vi "Excel Step Content test.vi"() -> ()   [LabVIEW 2019]
uses:
  Ctrl/ProjectStepSelect.ctl
  Global/Process Global.vi
panel:
  out "error out":errorcluster
  out "receive string":string
  out "concatenated string":string
  out "step content":string[](array[string])
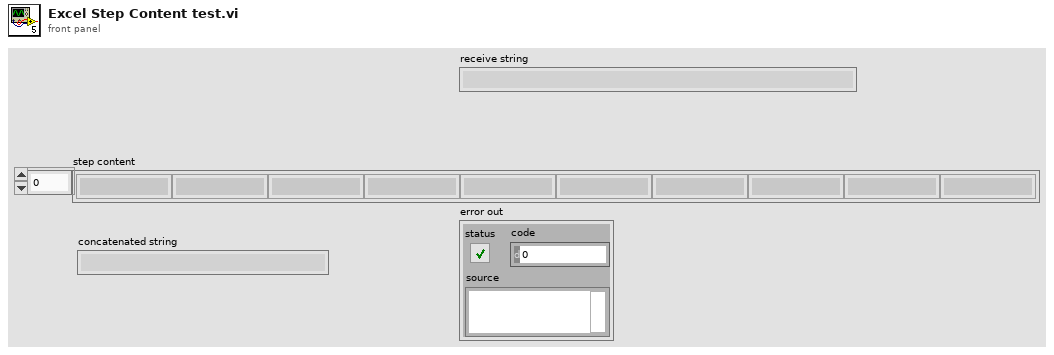
[diagram p1: front panel]
types:
  T1 = enum16{"Initial", "load", "read", "write", "write sn", "save"}
  T2 = enum16{"ProjectName", "Name", "Initial", "Reset", "Format", "Program1", "Program2", "Scan"}[]
  T3 = typedef "ProjectStepSelect.ctl" = enum16{"ProjectName", "Name", "Initial", "Reset", "Format", "Program1", "Program2", "Scan", "Finish", "MToolWork", "DataCheck", "DataSave", "OutputPLC", "WaitInputS1", "WaitInputOff"}
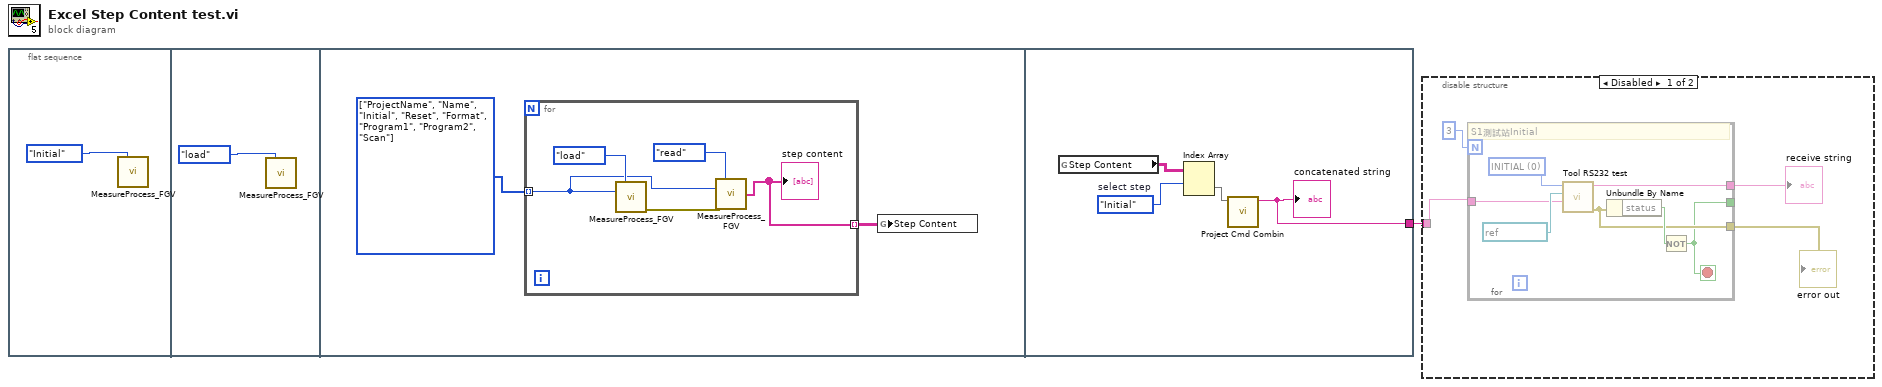
[diagram p0: block diagram]
diagram:
  n1 = flat-sequence {
    tunnel: [w11] -> w1
    frame #0 {
      n2 = call "MeasureProcess_FGV.vi"("action"=T1."Initial") -> ()  [unwired: 10 in, 5 out]
    }
    frame #1 {
      n3 = call "MeasureProcess_FGV.vi"("action"=T1."load") -> ()  [unwired: 10 in, 5 out]
    }
    frame #2 {
      w5 = T2 [enum."ProjectName", enum."Name", enum."Initial", enum."Reset", enum."Format", enum."Program1", enum."Program2", enum."Scan"] items=["ProjectName", "Name", "Initial", "Reset", "Format", "Program1", "Program2", "Scan"]
      n4 = for {
        tunnel: w5 -> [w7] mode=indexing
        tunnel: [w6] -> w4 mode=indexing
        n5 = call "MeasureProcess_FGV.vi"("action"=T1."load", "ProjectAct step"=w7) -> ("error out"=w8:errorcluster)  [unwired: 9 in, 4 out]
        n6 = call "MeasureProcess_FGV.vi"("action"=T1."read", "ProjectAct step"=w7, "error in"=w8) -> ("step content"=w6:string[])  [unwired: 8 in, 4 out]
        "step content" <- w6
      }
      n7 = global write "Process Global.vi" "Step Content"(w4) -> ()
    }
    frame #3 {
      w12 = ProjectStepSelect."Initial"  # select step
      n8 = global read "Process Global.vi" "Step Content"() -> (w14:string[][])
      n9 = Index Array(array=w14, index (row)=w12) -> (element=w13:string[])  [unwired: 1 in]
      n10 = call "Project Cmd Combin.vi"("Content Input"=w13) -> ("concatenated string"=w11:string)  [unwired: 8 in, 2 out]
      "concatenated string" <- w11
    }
  }
  n11 = disable-structure shown="Disabled" {
    disable-tunnel: w1 -> [w17 _]
    frame Disabled {
      n12 = for {
        N: 3 -> [_]
        tunnel: [w22] -> w16
        tunnel: [w21] -> w15
        tunnel: [w20] -> _
        tunnel: w17 -> [w19]
        stop <- w20 stop-if-true
        w24 = u16 0 items=["INITIAL", "RESET", "FORMAT", "PROGRAM1", "PROGRAM2", "FSKSCAN", "ASKSCAN"] ("action")
        # "S1測試站Initial"
        n13 = call "Tool RS232 test.vi"("Cmd In"=w19, "VISA resource name"=refnum<visa-resource-name> "COM3", "action"=w24) -> ("error out"=w21:errorcluster, "receive string"=w22:string)  [unwired: 7 in]
        n14 = Unbundle By Name(w21) -> ("status"=w25:bool)
        n15 = Not(x=w25) -> (.not. x?=w20:bool)
      }
      "receive string" <- w16
      "error out" <- w15
    }
    frame Enabled {
    }
  }
